vi "DS402 Drive - Get ECAT IOVar Data.vi"(6 "DS402 IOV In":T1, 8 "error in (no error)":errorcluster caption="Error in (no error)", 10 "ECAT IO Variable In":refnum<k21>[](array[refnum]), 11 "VS ref":T7=18446744073709551615 format="%.0x") -> (0 "Error out":errorcluster caption="Error Out", 1 "I/O Output Vars":T8[](array[typedef]) {"VS ref" format="%.0x"}, 2 "I/O Input Vars":T8[](array[typedef]) {"VS ref" format="%.0x"}, 3 "VS ref 2":T7=18446744073709551615 format="%.0x", 4 "DS402 IOV Out":T1, 5 "I/O Output Data":T3 {"BD Refs"."Data Reference" format="%.0x"}, 7 "I/O Input Data":T6 {"BD Refs"."Data Reference" format="%.0x"})   [LabVIEW 2016, in "Scan Engine Custom Device.lvlib"]
uses:
  Scan Engine Custom Device.lvlib
  Type Defs/DS402 Drive ECAT Slave IOV Cluster.ctl
  <vilib>/NI Veristand/Custom Device API/Custom Device Item Ref.ctl
  Type Defs/UDV Data Type.ctl
  Type Defs/Input Data.ctl
  <vilib>/NI Veristand/Custom Device API/Block Data Reference.ctl
  <vilib>/NI Veristand/Custom Device API/Data Reference.ctl
  Type Defs/Output Data.ctl
  Type Defs/DS402 Drive ECAT Slave Action IOV Cluster.ctl
  SVN/164039_TestCellStandardization/Source/DS402-SEECD/ECAT torque POC/Library/controls/state.ctl
  Type Defs/Data Ref FGV Command.ctl
  <vilib>/NI Veristand/Custom Device API/Data Access Type.ctl
  Globals/Property Strings.vi
  <vilib>/NI Veristand/Custom Device API/Custom Device API.lvlib
  <resource>/objmgr/ni.var.rc
  <vilib>/NI Veristand/Custom Device Tools/Custom Device Utility Library/Custom Device Utility Library.lvlib
  SVN/164039_TestCellStandardization/Source/DS402-SEECD/ECAT torque POC/Library/DS402.lvlib
panel:
  out "ECAT Variable Object out":refnum<k21>[](array[refnum])
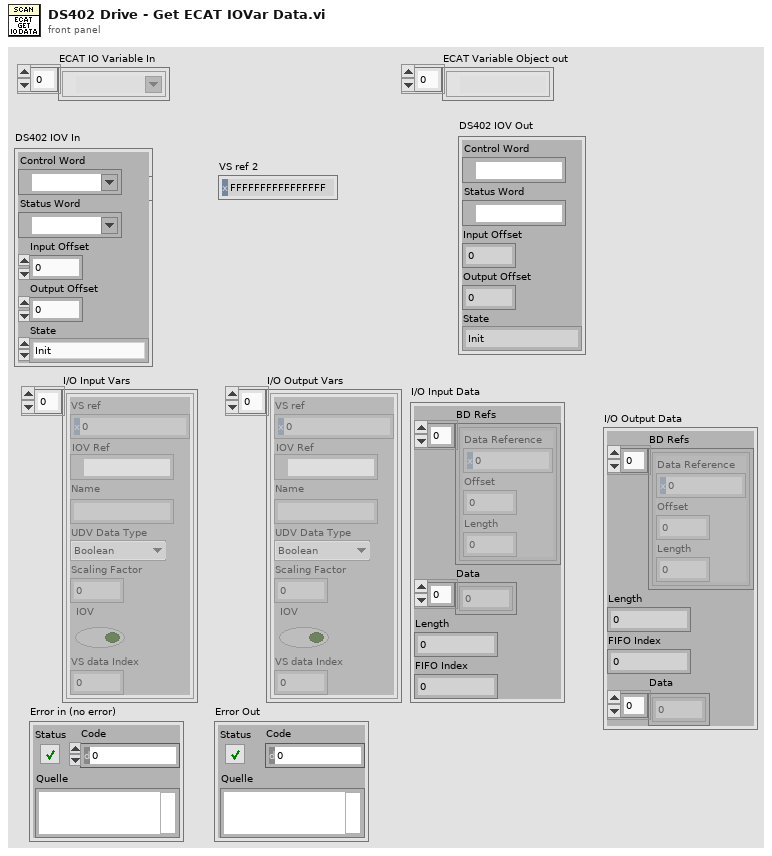
[diagram p1: front panel]
types:
  T1 = typedef "Scan Engine Custom Device.lvlib/DS402 Drive ECAT Slave Action IOV Cluster.ctl" = cluster{"Control Word":refnum<k21>, "Status Word":refnum<k21>, "Input Offset":i32, "Output Offset":i32, "State":T2}
  T2 = typedef "DS402.lvlib/state.ctl" = enum16{"Init", "Not Ready to Switch On", "Read Status Word", "Switch on disabled", "Ready to switch on", "Switched on", "Operation enabled", "Fault", "Fault reaction active", "Quick stop active", "Shutdown - Bad State", "Shutdown - Error", "Shutdown - Normal", "Shutdown - Fault"}
  T3 = typedef "Scan Engine Custom Device.lvlib/Output Data.ctl" = cluster{"BD Refs":T4[], "Length":i32, "FIFO Index":i32, "Data":dbl[]}
  T4 = typedef "Custom Device API.lvlib/Block Data Reference.ctl" = cluster{"Data Reference":T5, "Offset":u64, "Length":u64}
  T5 = typedef "Custom Device API.lvlib/Data Reference.ctl" = i32
  T6 = typedef "Scan Engine Custom Device.lvlib/Input Data.ctl" = cluster{"BD Refs":T4[], "Data":dbl[], "Length":i32, "FIFO Index":i32}
  T7 = typedef "Custom Device API.lvlib/Custom Device Item Ref.ctl" = u64
  T8 = typedef "Scan Engine Custom Device.lvlib/DS402 Drive ECAT Slave IOV Cluster.ctl" = cluster{"VS ref":T7, "IOV Ref":refnum<k21>, "Name":string, "UDV Data Type":T9, "Scaling Factor":dbl, "IOV":bool, "VS data Index":i32}
  T9 = typedef "Scan Engine Custom Device.lvlib/UDV Data Type.ctl" = enum16{"Boolean", "Fixed Point", "Int8", "Int16", "Int32", "Int64", "U32 Bit Field", "UInt8", "UInt16", "UInt32", "UInt64", "Other"}
  T10 = typedef "Scan Engine Custom Device.lvlib/Data Ref FGV Command.ctl" = enum16{"Intialize", "Get", "Update"}
  T11 = typedef "Custom Device API.lvlib/Data Access Type.ctl" = enum16{"Read", "Write"}
  T12 = typedef "Scan Engine Custom Device.lvlib/ECAT Channel Data Type.ctl" = enum16{"Boolean", "Fixed Point", "Int8", "Int16", "Int32", "Int64", "U32 Bit Field", "UInt8", "UInt16", "UInt32", "UInt64", "Other", "DBL"}
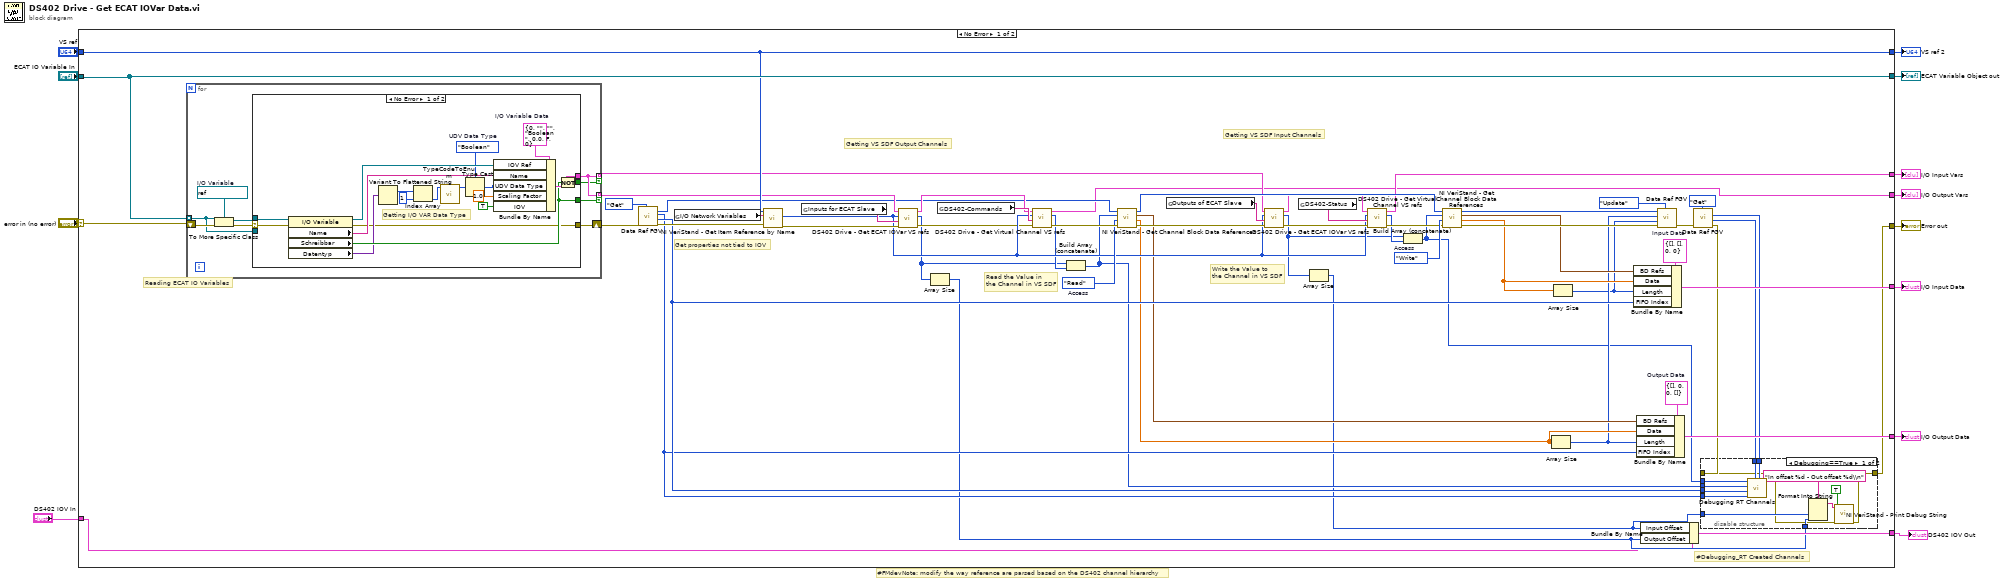
[diagram p0: block diagram]
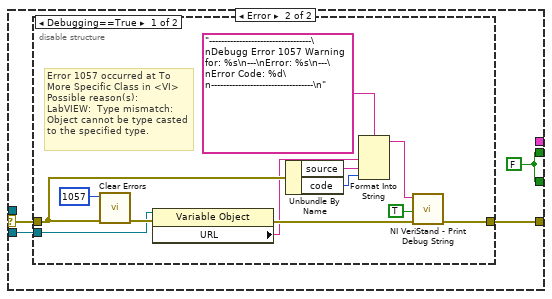
[diagram p2: hidden frame]
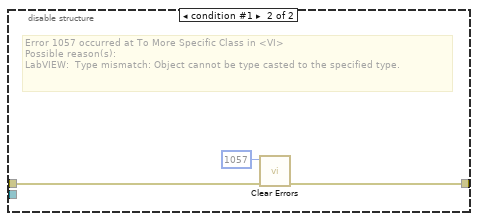
[diagram p3: hidden frame]
diagram:
  # "#FMdevNote: modify the way reference are parsed based on the DS402 channel hierarchy"
  n1 = case shown="No Error" "error in (no error)" {
    selector: "error in (no error)" -> [w31 w135]
    tunnel: "ECAT IO Variable In" -> [w71 w134]
    tunnel: [w52 w135] -> w10
    tunnel: [w71 w134] -> w9
    tunnel: "VS ref" -> [w68 w133]
    tunnel: [w22 _] -> w7
    tunnel: [w34 _] -> w6
    tunnel: [w68 w133] -> w5
    tunnel: [w65 _] -> w4
    tunnel: [w64 _] -> w3
    tunnel: "DS402 IOV In" -> [w13 w132]
    tunnel: [w30 w132] -> w1
    frame No Error {
      w40 = Data_Access_Type."Write"  # Access
      w45 = Data_Access_Type."Read"  # Access
      w66 = T3 {"BD Refs"=[], "Length"=0, "FIFO Index"=0, "Data"=[]}  # Output Data
      w67 = T6 {"BD Refs"=[], "Data"=[], "Length"=0, "FIFO Index"=0}  # Input Data
      # "Get properties not tied to IOV"
      # "#Debugging_RT Created Channels"
      # "Getting VS SDF Input Channels"
      # "Getting VS SDF Output Channels"
      # "Reading ECAT IO Variables"
      # "Write the Value to\nthe Channel in VS SDF"
      # "Read the Value in\nthe Channel in VS SDF"
      n2 = for {
        shift-right: [w75] -> w62
        shift-left: w31 -> [w74]
        tunnel: w71 -> [w72] mode=indexing
        tunnel: [w80] -> w37 mode=indexing if=w79
        tunnel: [w80] -> w49 mode=indexing if=w78
        w77 = refnum<k21> refnum  # I/O Variable
        n3 = To More Specific Class(target class=w77, reference=w72, error in=w74) -> (specific class reference=w76:refnum<k21>, error out=w73:errorcluster)
        n4 = case shown="No Error" w73 {
          selector: w73 -> [w83 w101]
          tunnel: [w96 _] -> w80
          tunnel: [w95 w102] -> w79
          tunnel: [w94 w102] -> w78
          tunnel: w76 -> [w93 _]
          tunnel: [w84 w100] -> w75
          tunnel: w72 -> [_ w99]
          frame No Error {
            w88 = UDV_Data_Type."Boolean"  # UDV Data Type
            w98 = T8 {"VS ref"=0, "IOV Ref"="", "Name"="", "UDV Data Type"=enum."Boolean", "Scaling Factor"=0.0, "IOV"=FALSE, "VS data Index"=0}  # I/O Variable Data
            # "Getting I/O VAR Data Type"
            n5 = property class="I/O Variable"(reference=w93, error in=w83) -> (reference out=w97:refnum<k21>, error out=w84:errorcluster, "Name"=w86:string, "Schreibbar"=w94:bool, "Datentyp"=w90:variant)
            n6 = Variant To Flattened String(Variant=w90) -> (1:w91:i16[])  [unwired: 1 out]
            n7 = Index Array(array=w91, index=1) -> (element=w89:i16)
            n8 = call "TypeCodeToEnum.vi"("Type Code (numbers in hexadecimal)"=w89) -> ("UDV Data Type"=w87:T12)  [unwired: 9 in, 1 out]
            n9 = Type Cast(type=w88, x=w87) -> (*(type *) &x=w85:T9)
            n10 = Bundle By Name(cluster=w98, "IOV Ref"=w97, "Name"=w86, "UDV Data Type"=w85, "Scaling Factor"=1.0, "IOV"=TRUE) -> (w96:T8)
            n11 = Not(x=w94) -> (.not. x?=w95:bool)
          }
          frame Error {
            w102 = FALSE
            n12 = disable-structure shown="Debugging==True" {
              disable-tunnel: w101 -> [w111 w116]
              disable-tunnel: [w108 w115] -> w100
              disable-tunnel: w99 -> [w107 _]
              frame condition #0 (active) {
                # "Error 1057 occurred at To More Specific Class in <VI>\nPossible reason(s):\nLabVIEW:  Type mismatch: Object cannot be type casted to the specified type."
                n13 = call <vilib>:"Clear Errors.vi"("error in (no error)"=w111, "specific error code to clear (0: all)"=1057) -> ("error out"=w110:errorcluster)  [unwired: 4 in, 1 out]
                n14 = property class="Variable Object"(reference=w107, error in=w110) -> (error out=w109:errorcluster, "URL"=w106:string)  [unwired: 1 out]
                n15 = Unbundle By Name(w111) -> ("source"=w105:string, "code"=w104:i32)
                n16 = Format Into String(format string="----------------------------------\nDebugg Error 1057 Warning for: %s\n---\nError: %s\n---\nError Code: %d\n----------------------------------\n" ("Format-String"), w106, w105, w104) -> (resulting string=w112:string)  [unwired: 2 in, 1 out]
                n17 = call <vilib>:"NI VeriStand - Print Debug String.vi"("error in (no error)"=w109, "Add to log file? (T)"=TRUE, "Message"=w112) -> ("error out"=w108:errorcluster)  [unwired: 8 in]
              }
              frame condition #1 {
                # "Error 1057 occurred at To More Specific Class in <VI>\nPossible reason(s):\nLabVIEW:  Type mismatch: Object cannot be type casted to the specified type."
                n18 = call <vilib>:"Clear Errors.vi"("error in (no error)"=w116, "specific error code to clear (0: all)"=1057) -> ("error out"=w115:errorcluster)  [unwired: 4 in, 1 out]
              }
            }
          }
        }
      }
      n19 = call "Data Ref FGV.vi"("Command"=Data_Ref_FGV_Command."Get", "error in (no error)"=w62) -> ("error out"=w61:errorcluster, "Output FIFO Index / Length"=w51:i32, "Input FIFO Index / Length"=w50:i32, "Device Ref out"=w29:T7)  [unwired: 6 in]
      n20 = global read "Property Strings.vi" "I/O Network Variables"() -> (w70:string)
      n21 = call <vilib>:"NI VeriStand - Get Item Reference by Name.vi"("error in (no error)"=w61, "Item Name"=w70, "Parent Ref in"=w68) -> ("error out"=w48:errorcluster, "Item Ref"=w36:T7)  [unwired: 5 in, 2 out]
      n22 = global read "Property Strings.vi" "Inputs for ECAT Slave"() -> (w59:string)
      n23 = call "DS402 Drive - Get ECAT IOVar VS refs.vi"("Fehler (Eingang, kein Fehler)"=w48, "Section Name"=w59, "Item Ref"=w36, "I/O Variable Data in"=w49) -> ("Fehler (Ausgang)"=w28:errorcluster, "Channel Refs"=w17:T7[], "I/O Variable Data out"=w44:T8[])  [unwired: 5 in]
      n24 = Array Size(array=w17) -> (size(s)=w14:i32)
      n25 = global read "Property Strings.vi" "DS402-Commands"() -> (w47:string)
      n26 = call "DS402 Drive - Get Virtual Channel VS refs.vi"("Fehler (Eingang, kein Fehler)"=w28, "Section Name"=w47, "Item Ref"=w36, "I/O Variable Data in"=w44) -> ("Fehler (Ausgang)"=w46:errorcluster, "Channel Refs"=w27:T7[], "I/O Variable Data out"=w22:T8[])  [unwired: 5 in]
      n27 = Build Array (concatenate)(w17, w27) -> (w18:T7[])
      n28 = call <vilib>:"NI VeriStand - Get Channel Block Data References.vi"("error in (no error)"=w46, "Access"=w45, "Channel Refs"=w18, "Device Ref in"=w29) -> ("error out"=w42:errorcluster, "Values Array"=w23:dbl[], "Block Data Refs"=w26:T4[], "Device Ref out"=w43:T7)  [unwired: 4 in]
      n29 = global read "Property Strings.vi" "Outputs of ECAT Slave"() -> (w58:string)
      n30 = call "DS402 Drive - Get ECAT IOVar VS refs.vi"("Fehler (Eingang, kein Fehler)"=w42, "Section Name"=w58, "Item Ref"=w36, "I/O Variable Data in"=w37) -> ("Fehler (Ausgang)"=w69:errorcluster, "Channel Refs"=w16:T7[], "I/O Variable Data out"=w35:T8[])  [unwired: 5 in]
      n31 = global read "Property Strings.vi" "DS402-Status"() -> (w41:string)
      n32 = Array Size(array=w16) -> (size(s)=w15:i32)
      n33 = call "DS402 Drive - Get Virtual Channel VS refs.vi"("Fehler (Eingang, kein Fehler)"=w69, "Section Name"=w41, "Item Ref"=w36, "I/O Variable Data in"=w35) -> ("Fehler (Ausgang)"=w39:errorcluster, "Channel Refs"=w25:T7[], "I/O Variable Data out"=w34:T8[])  [unwired: 5 in]
      n34 = Build Array (concatenate)(w16, w25) -> (w19:T7[])
      n35 = call <vilib>:"NI VeriStand - Get Channel Block Data References.vi"("error in (no error)"=w39, "Access"=w40, "Channel Refs"=w19, "Device Ref in"=w43) -> ("error out"=w38:errorcluster, "Values Array"=w24:dbl[], "Block Data Refs"=w32:T4[], "Device Ref out"=w33:T7)  [unwired: 4 in]
      n36 = Array Size(array=w23) -> (size(s)=w21:i32)
      n37 = Array Size(array=w24) -> (size(s)=w20:i32)
      n38 = Bundle By Name(cluster=w67, "BD Refs"=w32, "Data"=w24, "Length"=w20, "FIFO Index"=w51) -> (w65:T6)
      n39 = Bundle By Name(cluster=w66, "BD Refs"=w26, "Data"=w23, "Length"=w21, "FIFO Index"=w50) -> (w64:T3)
      n40 = Bundle By Name(cluster=w13, "Input Offset"=w15, "Output Offset"=w14) -> (w30:T1)
      n41 = call "Data Ref FGV.vi"("Command"=Data_Ref_FGV_Command."Update", "error in (no error)"=w38, "Output Length"=w20, "Input Length"=w21, "Device Ref in"=w33) -> ("error out"=w57:errorcluster)  [unwired: 3 in, 3 out]
      n42 = call "Data Ref FGV.vi"("Command"=Data_Ref_FGV_Command."Get", "error in (no error)"=w57) -> ("error out"=w53:errorcluster, "Output FIFO Index / Length"=w55:i32, "Input FIFO Index / Length"=w54:i32)  [unwired: 6 in, 1 out]
      n43 = disable-structure shown="Debugging==True" {
        disable-tunnel: w19 -> [w130 _]
        disable-tunnel: w18 -> [w129 _]
        disable-tunnel: w55 -> [w128 _]
        disable-tunnel: w54 -> [w127 _]
        disable-tunnel: w53 -> [w118 w131]
        disable-tunnel: [w124 w131] -> w52
        disable-tunnel: w50 -> [w126 _]
        disable-tunnel: w51 -> [w125 _]
        disable-tunnel: w15 -> [w122 _]
        disable-tunnel: w14 -> [w121 _]
        frame condition #0 (active) {
          n44 = call "Debugging RT Channels.vi"("Output FIFO Length"=w127, "Input FIFO Length"=w128, "Output FIFO Index"=w126, "Input FIFO Index"=w125, "Output  Channel Refs"=w129, "Input Channel Refs"=w130) -> ()  [unwired: 6 in]
          n45 = Format Into String(format string="In offset %d - Out offset %d\\n", w122, w121) -> (resulting string=w123:string)  [unwired: 2 in, 1 out]
          n46 = call <vilib>:"NI VeriStand - Print Debug String.vi"("error in (no error)"=w118, "Add to log file? (T)"=TRUE, "Message"=w123) -> ("error out"=w124:errorcluster)  [unwired: 8 in]
        }
        frame condition #1 {
        }
      }
    }
    frame Error {
    }
  }
  "I/O Input Vars" <- w6
  "I/O Output Vars" <- w7
  "Error out" <- w10
  "ECAT Variable Object out" <- w9
  "VS ref 2" <- w5
  "I/O Input Data" <- w4
  "I/O Output Data" <- w3
  "DS402 IOV Out" <- w1
